vi "Lockin.Mixer.vi"(8 "error in (no error)":errorcluster, 11 "Instrument.DAQ":refnum<class "Instrument.DAQ.lvclass">) -> (0 "error out":errorcluster, 3 "Instrument.DAQ":refnum<class "Instrument.DAQ.lvclass">)   [LabVIEW 2019, in "Instrument.Lockin.lvlib" / "Instrument.DAQ.lvclass"]
uses:
  Instrument.DAQ.lvclass
  Instrument.DAQ.lvclass/Instrument.DAQ.ctl
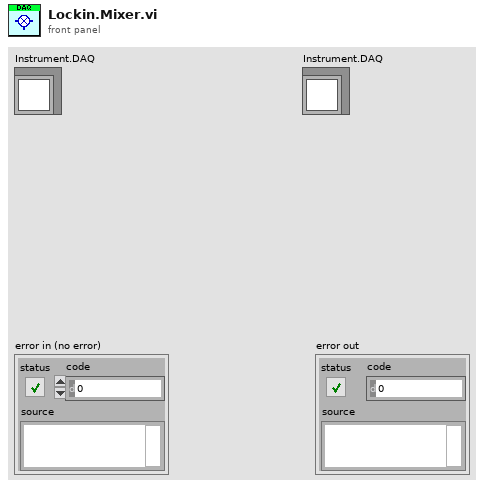
[diagram p1: front panel]
types:
  T1 = typedef "Instrument.Lockin.lvlib/Instrument.DAQ.lvclass/AI.Channel--Cluster--Array.ctl" = T2[]
  T2 = typedef "Instrument.Lockin.lvlib/Instrument.DAQ.lvclass/AI.Channel--Cluster.ctl" = cluster{"Enable?":bool, "Channel":i32, "References":i32[]}
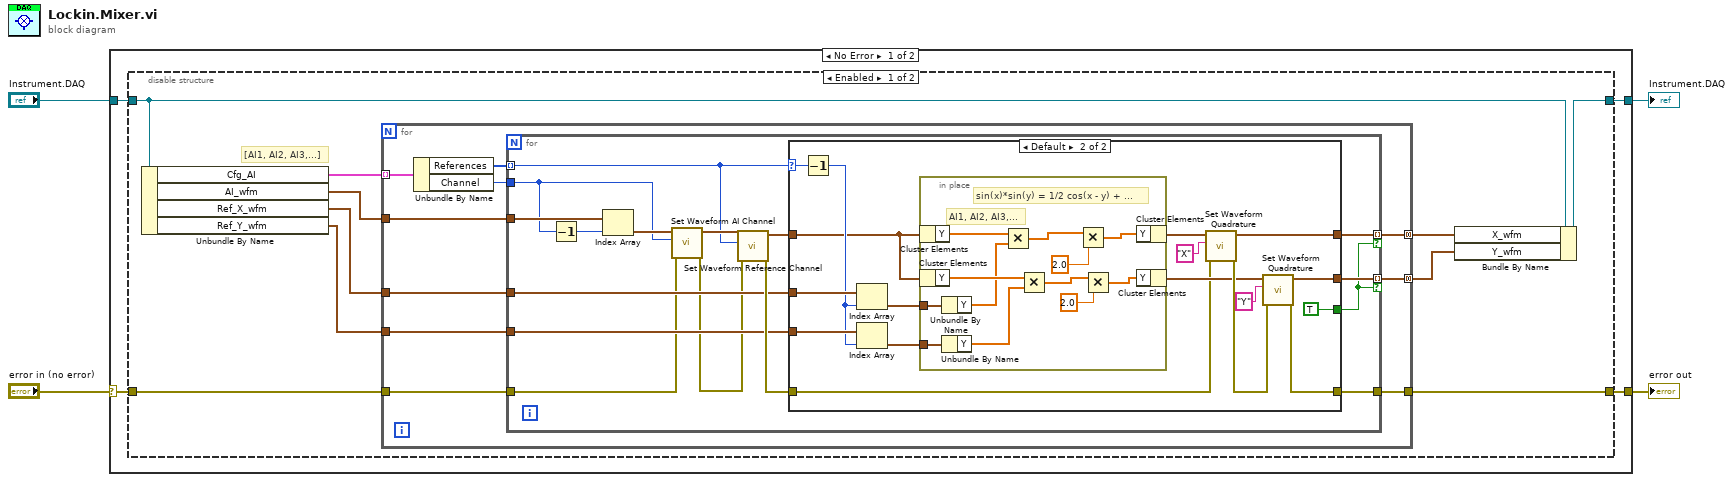
[diagram p0: block diagram]
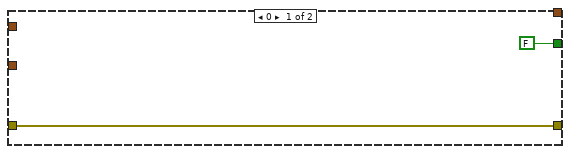
[diagram p2: hidden frame]
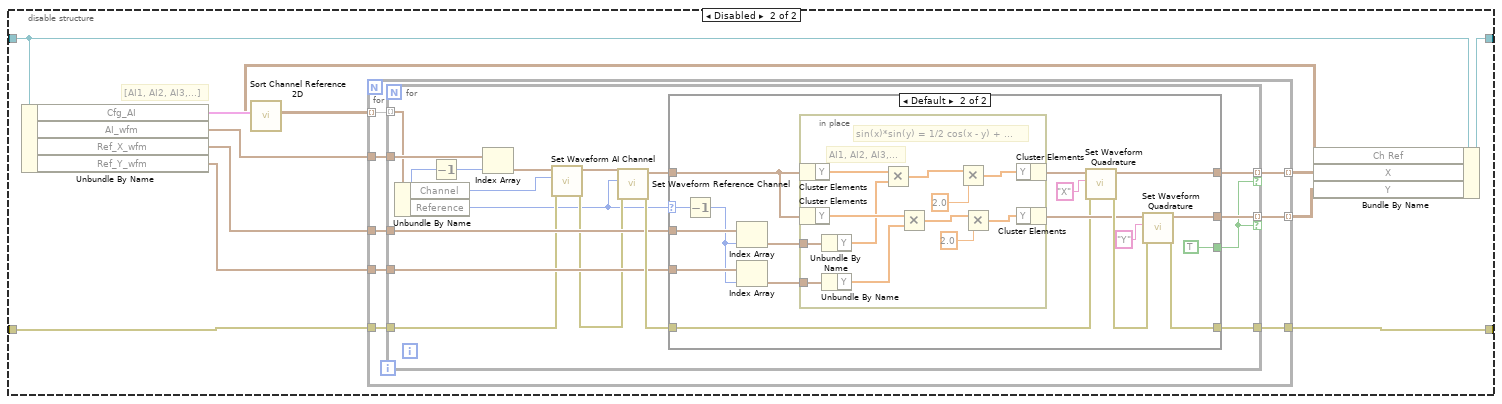
[diagram p3: hidden frame]
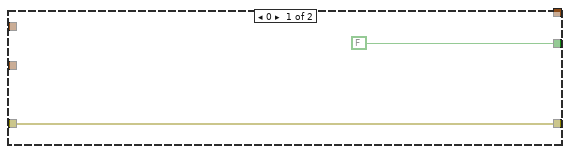
[diagram p4: hidden frame]
diagram:
  n1 = case shown="No Error" "error in (no error)" {
    selector: "error in (no error)" -> [w6 w144]
    tunnel: [w8 w144] -> w4
    tunnel: "Instrument.DAQ" -> [w7 w143]
    tunnel: [w5 w143] -> w2
    frame No Error {
      n2 = disable-structure shown="Enabled" {
        disable-tunnel: [w18 w86] -> w8
        disable-tunnel: w7 -> [w17 w85]
        disable-tunnel: w6 -> [w13 w81]
        disable-tunnel: [w10 w76] -> w5
        frame Enabled {
          # "[AI1, AI2, AI3,...]"
          n3 = Unbundle By Name(w17) -> ("Cfg_AI"=w9:T1, "AI_wfm"=w16:waveform(dbl)[], "Ref_X_wfm"=w15:waveform(dbl)[], "Ref_Y_wfm"=w14:waveform(dbl)[])
          n4 = for {
            tunnel: [w27] -> w12 mode=concatenating
            tunnel: w16 -> [w23]
            tunnel: w9 -> [w21] mode=indexing
            tunnel: w15 -> [w26]
            tunnel: w14 -> [w25]
            tunnel: [w24] -> w11 mode=concatenating
            tunnel: w13 -> [w22]
            tunnel: [w28] -> w18
            n5 = Unbundle By Name(w21) -> ("References"=w20:i32[], "Channel"=w19:i32)
            n6 = for {
              tunnel: [w41] -> w27 mode=indexing if=w37
              tunnel: w26 -> [w40]
              tunnel: w25 -> [w39]
              tunnel: [w38] -> w24 mode=indexing if=w37
              tunnel: w23 -> [w35]
              tunnel: w22 -> [w31]
              tunnel: [w44] -> w28
              tunnel: w20 -> [w30] mode=indexing
              tunnel: w19 -> [w29]
              n7 = Decrement(x=w29) -> (x-1=w33:i32)
              n8 = Index Array(array=w35, index=w33) -> (element=w36:waveform(dbl))
              n9 = call "Set Waveform AI Channel.vi"("error in (no error)"=w31, "AI Channel"=w29, "Waveform in"=w36) -> ("error out"=w32:errorcluster, "Waveform out"=w34:waveform(dbl))  [unwired: 7 in]
              n10 = call "Set Waveform Reference Channel.vi"("error in (no error)"=w32, "Reference Ch"=w30, "Waveform in"=w34) -> ("error out"=w42:errorcluster, "Waveform out"=w43:waveform(dbl))  [unwired: 7 in]
              n11 = case shown="Default" w30 {
                selector: w30 -> [_ w60]
                tunnel: [w46 w58] -> w44
                tunnel: w43 -> [_ w47]
                tunnel: w42 -> [w46 w49]
                tunnel: [_ w50] -> w41
                tunnel: [FALSE TRUE] -> w37
                tunnel: w40 -> [_ w62]
                tunnel: w39 -> [_ w61]
                tunnel: [_ w48] -> w38
                frame 0 {
                }
                frame Default {
                  n12 = Decrement(x=w60) -> (x-1=w55:i32)
                  n13 = Index Array(array=w62, index=w55) -> (element=w54:waveform(dbl))
                  n14 = Index Array(array=w61, index=w55) -> (element=w53:waveform(dbl))
                  n15 = in-place {
                    in-place-border: w54 -> [w73]
                    in-place-border: w53 -> [w71]
                    # "sin(x)*sin(y) = 1/2 cos(x - y) + ..."
                    # "AI1, AI2, AI3,..."
                    n16 = in-place-cluster #1(w47) -> ("Y"=w75:dbl[])
                    n17 = in-place-cluster #2(w47) -> ("Y"=w74:dbl[])
                    n18 = Unbundle By Name(w73) -> ("Y"=w72:dbl[])
                    n19 = Unbundle By Name(w71) -> ("Y"=w70:dbl[])
                    n20 = Multiply(x=w75, y=w72) -> (x*y=w69:dbl[])
                    n21 = Multiply(x=w74, y=w70) -> (x*y=w68:dbl[])
                    n22 = Multiply(x=w69, y=2.0) -> (x*y=w66:dbl[])
                    n23 = Multiply(x=w68, y=2.0) -> (x*y=w67:dbl[])
                    n24 = in-place-cluster #1("Y"=w66) -> (w51:waveform(dbl))
                    n25 = in-place-cluster #2("Y"=w67) -> (w52:waveform(dbl))
                  }
                  n26 = call "Set Waveform Quadrature.vi"("error in (no error)"=w49, "Quadratude"="X", "Waveform in"=w51) -> ("error out"=w59:errorcluster, "Waveform out"=w50:waveform(dbl))  [unwired: 7 in]
                  n27 = call "Set Waveform Quadrature.vi"("error in (no error)"=w59, "Quadratude"="Y", "Waveform in"=w52) -> ("error out"=w58:errorcluster, "Waveform out"=w48:waveform(dbl))  [unwired: 7 in]
                }
              }
            }
          }
          n28 = Bundle By Name(cluster=w17, "X_wfm"=w12, "Y_wfm"=w11) -> (w10:refnum<class "Instrument.DAQ.lvclass">)
        }
        frame Disabled {
          # "[AI1, AI2, AI3,...]"
          n29 = Unbundle By Name(w85) -> ("Cfg_AI"=w78:T1, "AI_wfm"=w84:waveform(dbl)[], "Ref_X_wfm"=w83:waveform(dbl)[], "Ref_Y_wfm"=w82:waveform(dbl)[])
          n30 = call "Sort Channel Reference 2D.vi"("Cfg.AI"=w78) -> ("Channel Reference 2D"=w77:cluster{"Channel":i32, "Reference":i32}[][])  [unwired: 10 in]
          n31 = for {
            tunnel: [w93] -> w80 mode=indexing
            tunnel: w84 -> [w88]
            tunnel: w77 -> [w89] mode=indexing
            tunnel: w83 -> [w92]
            tunnel: w82 -> [w91]
            tunnel: [w90] -> w79 mode=indexing
            tunnel: w81 -> [w87]
            tunnel: [w94] -> w86
            n32 = for {
              tunnel: w89 -> [w100] mode=indexing
              tunnel: [w108] -> w93 mode=indexing if=w104
              tunnel: w92 -> [w107]
              tunnel: w91 -> [w106]
              tunnel: [w105] -> w90 mode=indexing if=w104
              tunnel: w88 -> [w102]
              tunnel: w87 -> [w96]
              tunnel: [w111] -> w94
              n33 = Unbundle By Name(w100) -> ("Channel"=w98:i32, "Reference"=w95:i32)
              n34 = Decrement(x=w98) -> (x-1=w99:i32)
              n35 = Index Array(array=w102, index=w99) -> (element=w103:waveform(dbl))
              n36 = call "Set Waveform AI Channel.vi"("error in (no error)"=w96, "AI Channel"=w98, "Waveform in"=w103) -> ("error out"=w97:errorcluster, "Waveform out"=w101:waveform(dbl))  [unwired: 7 in]
              n37 = call "Set Waveform Reference Channel.vi"("error in (no error)"=w97, "Reference Ch"=w95, "Waveform in"=w101) -> ("error out"=w109:errorcluster, "Waveform out"=w110:waveform(dbl))  [unwired: 7 in]
              n38 = case shown="Default" w95 {
                selector: w95 -> [_ w127]
                tunnel: [w113 w125] -> w111
                tunnel: w110 -> [_ w114]
                tunnel: w109 -> [w113 w116]
                tunnel: [_ w117] -> w108
                tunnel: [FALSE TRUE] -> w104
                tunnel: w107 -> [_ w129]
                tunnel: w106 -> [_ w128]
                tunnel: [_ w115] -> w105
                frame 0 {
                }
                frame Default {
                  n39 = Decrement(x=w127) -> (x-1=w122:i32)
                  n40 = Index Array(array=w129, index=w122) -> (element=w121:waveform(dbl))
                  n41 = Index Array(array=w128, index=w122) -> (element=w120:waveform(dbl))
                  n42 = in-place {
                    in-place-border: w121 -> [w140]
                    in-place-border: w120 -> [w138]
                    # "sin(x)*sin(y) = 1/2 cos(x - y) + ..."
                    # "AI1, AI2, AI3,..."
                    n43 = in-place-cluster #3(w114) -> ("Y"=w142:dbl[])
                    n44 = in-place-cluster #4(w114) -> ("Y"=w141:dbl[])
                    n45 = Unbundle By Name(w140) -> ("Y"=w139:dbl[])
                    n46 = Unbundle By Name(w138) -> ("Y"=w137:dbl[])
                    n47 = Multiply(x=w142, y=w139) -> (x*y=w136:dbl[])
                    n48 = Multiply(x=w141, y=w137) -> (x*y=w135:dbl[])
                    n49 = Multiply(x=w136, y=2.0) -> (x*y=w133:dbl[])
                    n50 = Multiply(x=w135, y=2.0) -> (x*y=w134:dbl[])
                    n51 = in-place-cluster #3("Y"=w133) -> (w118:waveform(dbl))
                    n52 = in-place-cluster #4("Y"=w134) -> (w119:waveform(dbl))
                  }
                  n53 = call "Set Waveform Quadrature.vi"("error in (no error)"=w116, "Quadratude"="X", "Waveform in"=w118) -> ("error out"=w126:errorcluster, "Waveform out"=w117:waveform(dbl))  [unwired: 7 in]
                  n54 = call "Set Waveform Quadrature.vi"("error in (no error)"=w126, "Quadratude"="Y", "Waveform in"=w119) -> ("error out"=w125:errorcluster, "Waveform out"=w115:waveform(dbl))  [unwired: 7 in]
                }
              }
            }
          }
          n55 = Bundle By Name(cluster=w85, "Ch Ref"=w77, "X"=w80, "Y"=w79) -> (w76:refnum<class "Instrument.DAQ.lvclass">)
        }
      }
    }
    frame Error {
    }
  }
  "error out" <- w4
  "Instrument.DAQ" <- w2
